vi "WPs and Obstacles 8.vi"(7 "sim path":path, 8 "Mode":bool, 9 "WP Real Longs":dbl[](array[numeric])=[81.2671, 81.26711, 81.267112, 81.267332, 81.267916, 81.267137, 81.267874, 81.267301, 81.267913, 81.26772] format="%#_8g", 10 "WP Real Lats":dbl[](array[numeric])=[37.1528, 37.15281, 37.152877, 37.152903, 37.152565, 37.152792, 37.152806, 37.152779, 37.152868, 37.152484] format="%#_8g") -> (1 "WP Lats and Longs":cluster{"WP Lats":dbl[], "WP Longs":dbl[]} {"WP Longs" format="%#_8g"; "WP Lats" format="%#_8g"}, 2 "Sim Matrx":u8[][](array[numeric]), 3 "WP Map":cluster{"WP Longs":dbl[], "WP Lats":dbl[]}(graph), 4 "Sim Course":picture)   [LabVIEW 2014]
panel:
  out "WPl":dbl[](array[numeric]) format="%#_8g"
  out "WPL":dbl[](array[numeric]) format="%#_8g"
  out "nWPl":dbl[](array[numeric])
  out "nWPL":dbl[](array[numeric])
  out "num of wps":dbl
  in  "Empty Array":dbl[][](array[numeric])
  in  "Empty 2D Picture":picture
  # "Waypoint and Obstacles 8 (Uses Paint and On-Screen WPs)"
  # "Inputs:"
  # "20"
  # "Outputs:"
  # "Sim Painted Picture to matrix"
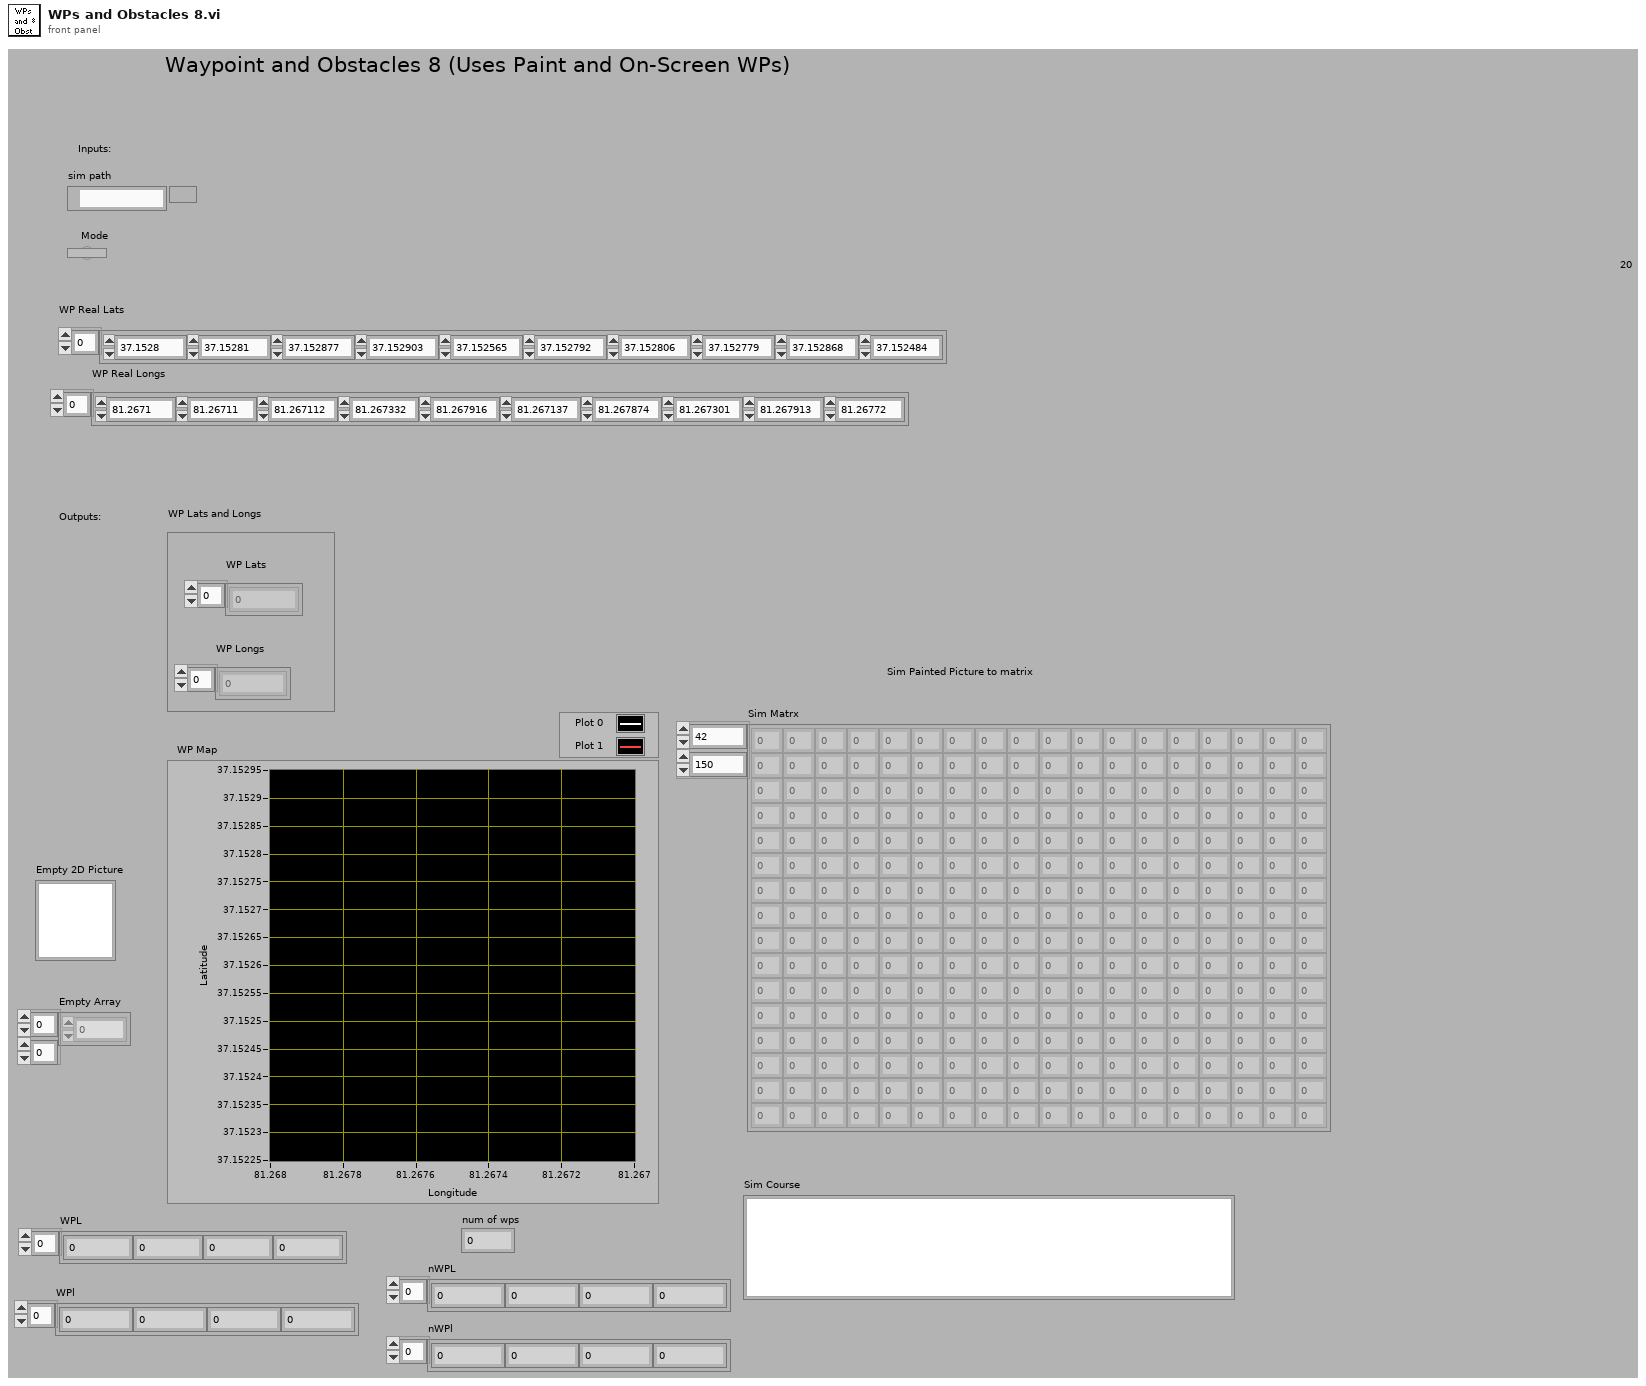
[diagram p1: front panel]
types:
  T1 = cluster{"WP Real Lats":dbl[], "WP Real Longs":dbl[]}
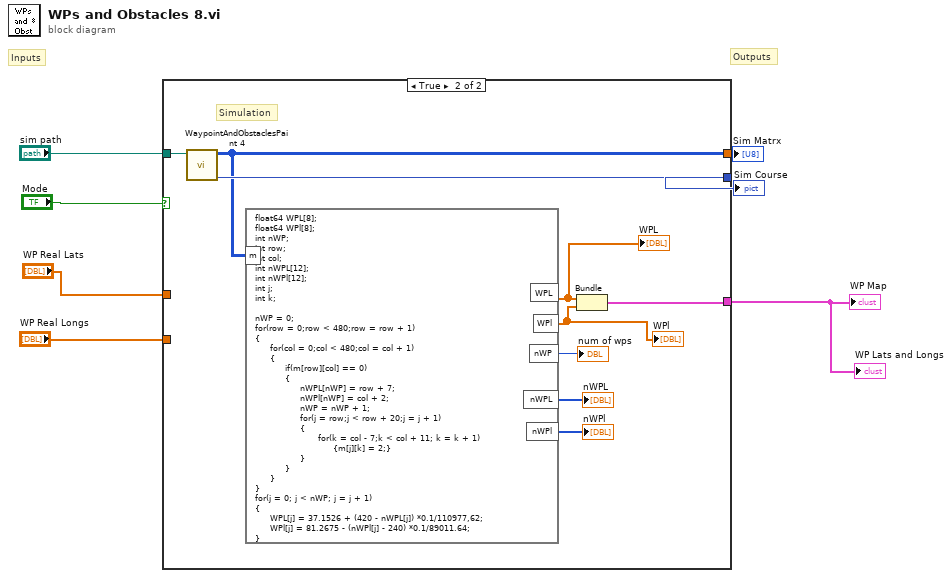
[diagram p0: block diagram]
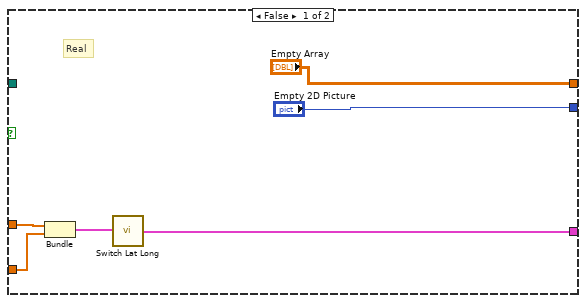
[diagram p2: hidden frame]
diagram:
  # "Inputs"
  # "Outputs"
  n1 = case shown="True" "Mode" {
    tunnel: "WP Real Lats" -> [w13 _]
    tunnel: "WP Real Longs" -> [w12 _]
    tunnel: "sim path" -> [_ w22]
    tunnel: ["Empty Array" w20] -> w3
    tunnel: ["Empty 2D Picture" w21] -> w2
    tunnel: [w8 w19] -> w1
    frame False {
      # "Real"
      n2 = Bundle("WP Real Lats"=w13, "WP Real Longs"=w12) -> (w9:T1)  [unwired: 1 in]
      n3 = call "Switch Lat Long.vi"("WP Lats and Longs for GIC"=w9) -> ("WP Lats and Longs switched"=w8:cluster{"WP Longs":dbl[], "WP Lats":dbl[]})
    }
    frame True {
      # "Simulation"
      n4 = call "WaypointAndObstaclesPaint 4.vi"("Sim Path"=w22) -> ("Sim Course"=w21:picture, 3:w20:u8[][])  [unwired: 9 in]
      n5 = formula code="float64 WPL[8];\nfloat64 WPl[8];\nint nWP;\nint row;\nint col;\nint nWPL[12];\nint nWPl[12];\nint j;\nint k;\n\nnWP = 0;\nfor(row = 0;row < 480;row = row + 1)\n{\n     for(col = 0;col < 480;col = col + 1)\n     {\n          if(m[row][col] == 0)\n          {     \n               nWPL[nWP] = row + 7;\n               nWPl[nWP] = col + 2; \n               nWP = nWP + 1;\n               for(j = row;j < row + 20;j = j + 1)\n               {\n                     for(k = col - 7;k < col + 11; k = k + 1)\n                          {m[j][k] = 2;}\n               }\n          }    \n     }\n}\nfor(j = 0; j < nWP; j = j + 1)\n{\n     WPL[j] = 37.1526 + (420 - nWPL[j]) *0.1/110977,62;\n     WPl[j] = 81.2675 - (nWPl[j] - 240) *0.1/89011.64;\n}"("m"=w20) -> ("WPL"=w15:dbl[], "WPl"=w14:dbl[], "nWP"=→"num of wps":i32, "nWPL"=→"nWPL":i32[], "nWPl"=→"nWPl":i32[])
      "WPL" <- w15
      "WPl" <- w14
      n6 = Bundle(w15, w14) -> (w19:cluster{dbl[], dbl[]})  [unwired: 1 in]
    }
  }
  "WP Lats and Longs" <- w1
  "Sim Matrx" <- w3
  "Sim Course" <- w2
  "WP Map" <- w1
